vi "Basement HMI.vi"() -> ()   [LabVIEW 2018]
uses:
  <vilib>/NI/Current Value Table/Type Defs/Single Tag.ctl
  <vilib>/NI/Current Value Table/Type Defs/Data Types.ctl
  <vilib>/Utility/sysdir.llb/System Directory Type.ctl
  <vilib>/NI/Current Value Table/DataTypes/Boolean_Write.vi
  <vilib>/NI/STM/TCP/Read Meta Data (TCP Ref).vi
  <vilib>/NI/STM/TCP/Get Connection Reference (TCP).vi
  <vilib>/NI/Current Value Table/Type to Enum.vi
  <vilib>/NI/Current Value Table/DataTypes/Boolean_Type To Enum.vi
  <vilib>/NI/AMC/Read Termination Message.vi
  <vilib>/NI/AMC/Create Single Message.vi
  <vilib>/NI/AMC/Update Message Routing Info.vi
  <vilib>/NI/STM/TCP/Read Meta Data (TCP Clst).vi
  <vilib>/NI/Current Value Table/FGVs/CVT Globals.vi
  <vilib>/NI/Current Value Table/FGVs/Tag Memory.vi
  <vilib>/NI/Current Value Table/Memory Block.vi
  <vilib>/NI/Current Value Table/DataTypes/Boolean_Memory Block.vi
  <vilib>/NI/AMC/Globals.vi
  <vilib>/NI/STM/TCP/Write Message (TCP).vi
  <vilib>/NI/AMC/Send Message.vi
  <vilib>/NI/AMC/AMC.lvlib
  <vilib>/NI/STM/NI STM.lvlib
  <vilib>/NI/Current Value Table/Current Value Table.lvlib
panel:
  out "status":string
  in  "Tab Control":T1(tab)
  in  "Reset Alarms":bool
  in  "Run":bool
  in  "exit":bool
  in  "Alarms":i32(listbox)=-1
  out "PLC Model":string
  out "PLC Firmware":string
  out "PLC Sweep Time":dbl format="%#.4f"
  out "Circulator 3":bool caption="Circulator P3"
  out "Chilled Water In":dbl(knob) scale=0.0..25.0
  out "Chilled Water Out":dbl(knob) scale=0.0..25.0
  out "Chilled Water Valve":dbl(slide) scale=0.0..100.0
  out "Tempered Water In":dbl(knob) scale=15.0..35.0
  out "Tempered Water Out":dbl(knob) scale=15.0..35.0
  out "Tempered Water Valve":dbl(slide) scale=0.0..100.0
  out "Circulator 1":bool caption="Circulator P1"
  out "Circulator 2":bool caption="Circulator P2"
  out "Boiler Water In":dbl(knob) scale=10.0..100.0
  out "Boiler Water Out":dbl(knob) scale=10.0..100.0
  out "Boiler Water Valve":dbl(slide) scale=0.0..100.0
  out "Oxide Left To Dose":dbl format="%#.1f"
  out "OxideDose Indicate 1":bool caption="Oxide Dosing"
  in  "Oxide grams to Add 1":dbl=2.0 caption="Oxide grams to Add" min=-1000.0 max=1000.0 step=0.1
  in  "Dose Extra Oxide 1":bool caption="Dose Extra Oxide"
  out "FlowToOxSys 1":dbl(slide) caption="Flow To Oxide Sys" scale=0.0..12.0 scale format="%.1f"
  out "Chilled Water Injection 1":u8(slide) caption="Chilled Water Injection" scale=0.0..100.0
  out "Tempered Water Injection 1":u8(slide) caption="Tempered Water Injection" scale=0.0..100.0
  in  "T Setpoint 1":dbl=15.0 caption="T Setpoint" min=15.0 max=28.0 step=0.5
  in  "Flow to Oxide 1":dbl=2.0 caption="Flow to Oxide" min=2.0 max=12.0 step=0.1
  in  "Enable Oxide System 1":bool caption="Enable Oxide System"
  in  "Enable T Control 1":bool caption="Enable T Control"
  out "T °C 1":dbl(slide) caption="T °C" scale=0.0..30.0
  out "Proc4MainPumpInd 2":bool
  out "DI Flow Rate 1":u8(slide) caption="DI Flow Rate" scale=0.0..75.0
  out "Liters DI Added 1":dbl caption="Liters DI Added" format="%.1f"
  in  "DI Add Volume 1":dbl caption="DI Add Volume" min=0.0 max=500.0 step=0.25
  in  "Add DI water 1":bool caption="Add DI Water"
  in  "Drain System to Tree 1":bool caption="Drain System to Tree"
  out "Plating Tanks In Use South PE":bool
  in  "Enable Main Pump":bool
  out "Tank 1":dbl(slide) caption="Tank" scale=0.0..1000.0
  out "Oxide Pump":bool
  out "Oxide Pump 2":bool
  out "FlowToOxSys 2":dbl(slide) caption="Flow To Oxide Sys" scale=0.0..12.0 scale format="%.1f"
  in  "DI Add Volume 2":dbl caption="DI Add Volume"
  in  "Add DI water 2":bool caption="Add DI Water"
  out "Chilled Water Injection2":u8(slide) caption="Chilled Water Injection" scale=0.0..100.0
  out "Tempered Water Injection2":u8(slide) caption="Tempered Water Injection" scale=0.0..100.0
  out "Proc2MainPumpInd":bool
  in  "T Setpoint 2":dbl caption="T Setpoint"
  out "DI Flow Rate 2":u8(slide) caption="DI Flow Rate" scale=0.0..100.0
  in  "Flow to Oxide 2":dbl caption="Flow to Oxide"
  in  "Enable Oxide System 2":bool caption="Enable Oxide System"
  in  "Enable T Control 2":bool caption="Enable T Control"
  out "Liters DI Added 2":dbl caption="Liters DI Added" format="%.1f"
  out "T °C 2":dbl(slide) caption="T °C" scale=0.0..30.0
  out "Plating Tanks In Use S. PE":bool
  in  "Drain System to Tree 2":bool caption="Drain System to Tree"
  in  "Enable Main Pump 2":bool caption="Enable Main Pump"
  out "Tank 2":dbl(slide) scale=0.0..1000.0
  out "Oxide Pump 3":bool
  in  "Flow to Oxide 3":dbl=2.0 caption="Flow to Oxide" min=2.0 max=12.0 step=0.10000000149011612 format="%.1f"
  in  "Enable Oxide System 3":bool caption="Enable Oxide System"
  out "Proc2MainPumpInd 2":bool
  in  "DI Add Volume 3":dbl caption="DI Add Volume"
  in  "Add DI water 3":bool caption="Add DI Water"
  in  "T Setpoint 3":dbl=15.0 caption="T Setpoint" min=15.0 max=85.0 step=0.1
  in  "Enable T Control 3":bool caption="Enable T Control"
  out "Chilled Water Injection2 3":u8(slide) caption="Boiler Water Injection" scale=0.0..100.0
  out "Chilled Water Injection2 2":u8(slide) caption="Chilled Water Injection" scale=0.0..100.0
  out "Tempered Water Injection2 2":u8(slide) caption="Tempered Water Injection" scale=0.0..100.0
  out "T °C 3":dbl(slide) caption="T °C" scale=0.0..100.0
  out "Tank 3":dbl(slide) scale=0.0..1000.0
  out "DI Flow Rate 3":u8(slide) caption="DI Flow Rate" scale=0.0..100.0
  out "Liters DI Added 3":dbl caption="Liters DI Added" format="%.1f"
  in  "Drain System to Tree 3":bool caption="Drain System to Tree"
  in  "Enable Main Pump 3":bool caption="Enable Main Pump"
  out "Plating Tanks In Use S. PE 3":bool caption="Plating Tanks In Use S. PE"
  out "FlowToOxSys 3":dbl(slide) caption="Flow To Oxide Sys" scale=0.0..12.0 scale format="%.1f"
  in  "Pump Speed 4":dbl=5.0 caption="Pump Speed" min=5.0 max=100.0 step=0.5
  out "Proc4MainPumpInd":bool
  out "DI Flow Rate 4":u8(slide) caption="DI Flow Rate" scale=0.0..75.0
  out "Liters DI Added 4":dbl caption="Liters DI Added" format="%.1f"
  in  "DI Add Volume 4":dbl caption="DI Add Volume"
  in  "Add DI water 4":bool caption="Add DI Water"
  in  "Drain System to Tree 4":bool caption="Drain System to Tree"
  in  "Enable Main Pump 4":bool caption="Enable Main Pump"
  out "Tank 340":dbl(slide) scale=0.0..1500.0
  # "°C"
  # "°C"
  # "°C"
  # "°C"
  # "°C"
  # "°C"
  # "T 341"
  # "T 345"
  # "T 349"
  # "%"
  # "T 340"
  # "L"
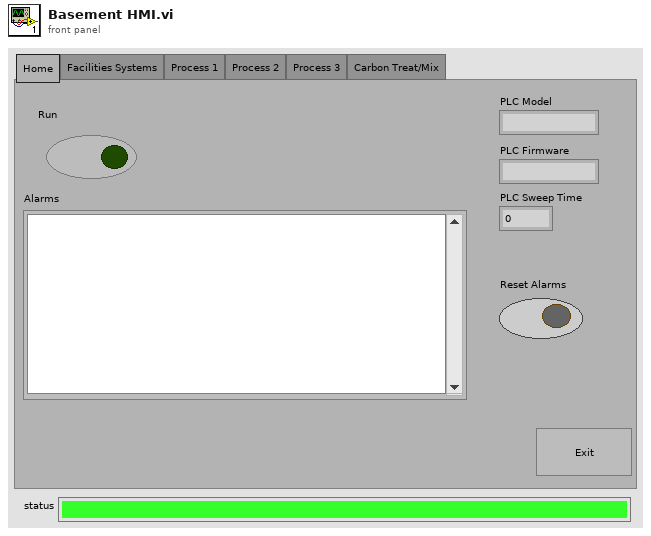
[diagram p1: front panel]
types:
  T1 = enum32{"Home", "Facilities Systems", "Process 1", "Process 2", "Process 3", "Carbon Treat/Mix"}
  T2 = typedef "System Directory Type.ctl" = i32
  T3 = typedef "Current Value Table.lvlib/Single Tag.ctl" = cluster{"Data Type":T4, "Name":string, "Value":string, "Description":string}
  T4 = typedef "Current Value Table.lvlib/Data Types.ctl" = enum16{"Double", "Single", "I64", "I32", "I16", "I8", "U64", "U32", "U16", "U8", "String", "Boolean", "Array of U8", "Array of U16", "Array of U32", "Array of U64", "Array of I64", "Array of I32", "Array of I16", "Array of I8", "Array of Double", "Array of Single", "Array of Boolean", "Array of String"}
  T5 = typedef "tae_AlarmTagConfiguration.ctl" = cluster{"Name":string, "DataType":T6, "Alarm Configuration":T7}
  T6 = typedef "cvt_Data Types.ctl" = enum16{"Bool", "U8", "I32", "Double", "String", "Enum"}
  T7 = typedef "tae_AlarmConfiguration.ctl" = cluster{"Type":T8, "High Level":dbl, "Low Level":dbl, "Hysterisis":dbl, "Deadband":dbl}
  T8 = typedef "tae_AlarmType.ctl" = enum32{"Bool True", "Bool False", "Over Limit", "Under Limit", "Out-of-Range", "Enum Equal", "Enum Not Equal"}
  T9 = typedef "Current Value Table.lvlib/File Format.ctl" = cluster{"Tags":T3[], "Group Listings":T10[]}
  T10 = typedef "Current Value Table.lvlib/Tag Grouping set.ctl" = cluster{"Group":string, "Tag Names":string[]}
  T11 = typedef "tae_AlarmCommOut.ctl" = refnum<queue>
  T12 = typedef "tae_AlarmTagList.ctl" = T5[]
  T13 = typedef "AMC.lvlib/Message Queue.ctl" = refnum<queue>
  T14 = typedef "NI STM.lvlib/TCP Connection Info.ctl" = cluster{"connection ID":refnum<k5>, "meta data":T15[]}
  T15 = typedef "NI STM.lvlib/MetaDataElement.ctl" = string
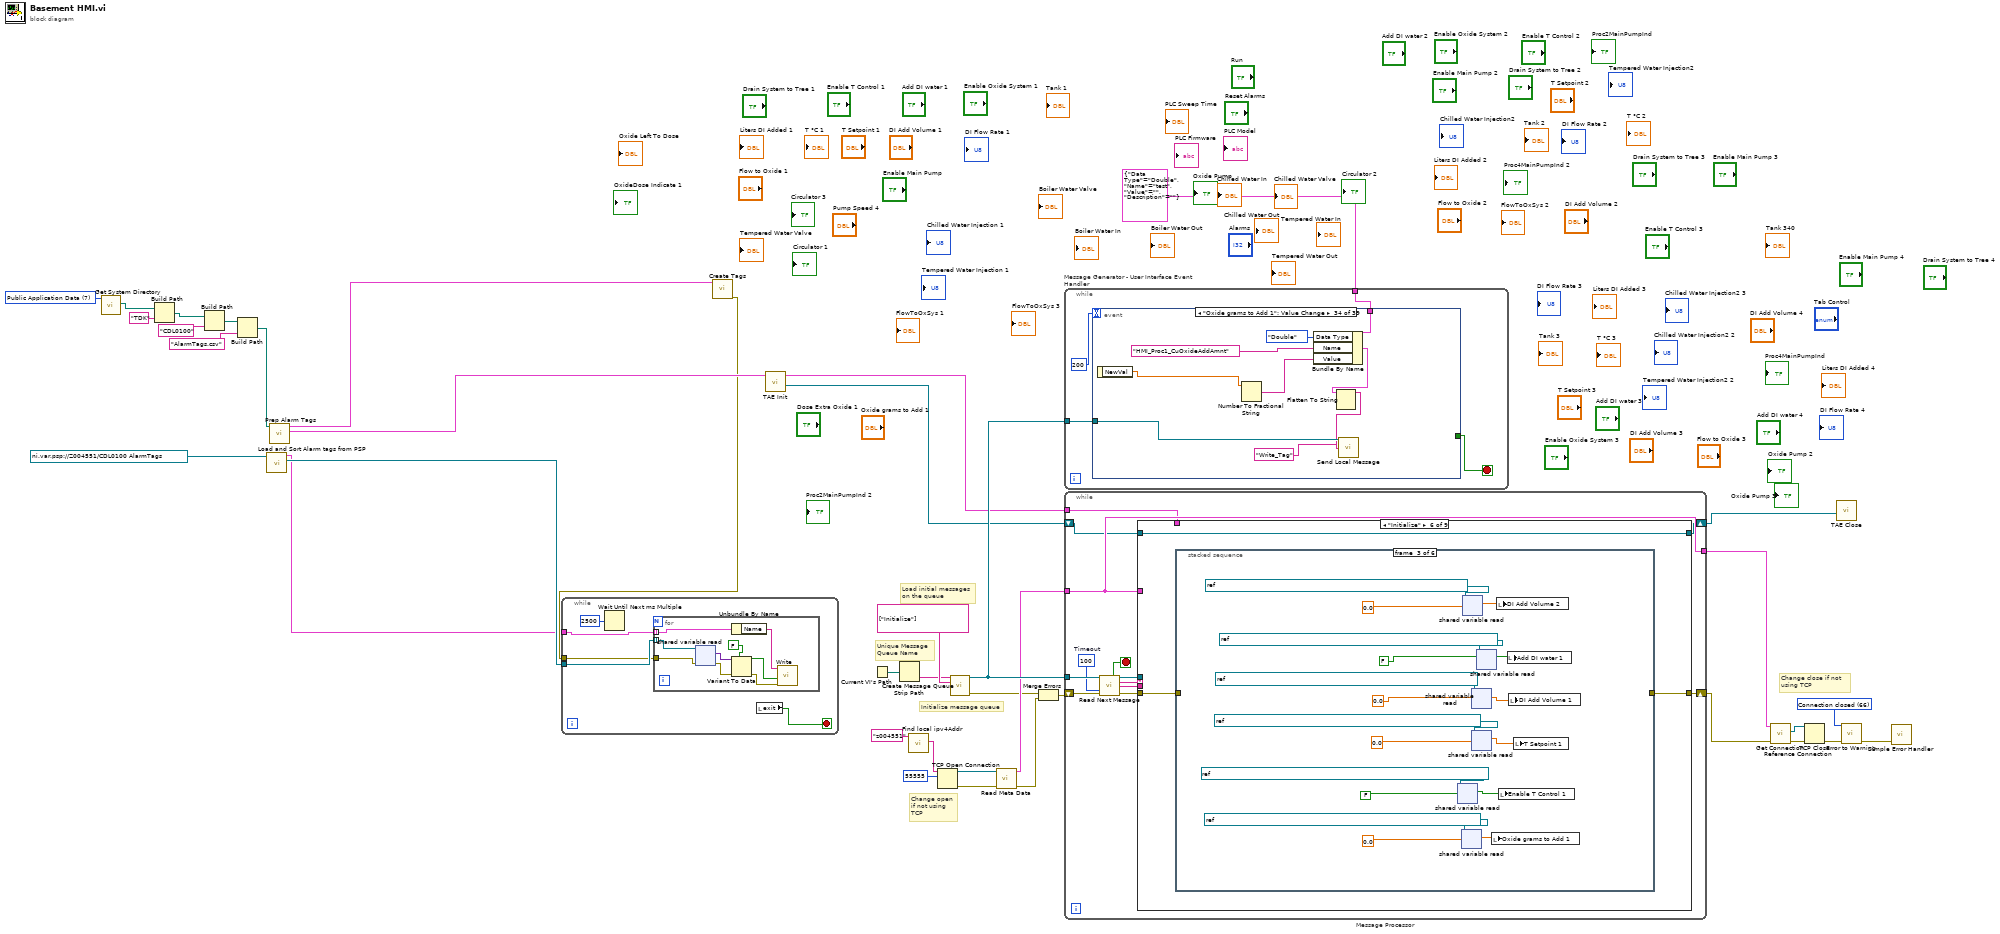
[diagram p0: block diagram]
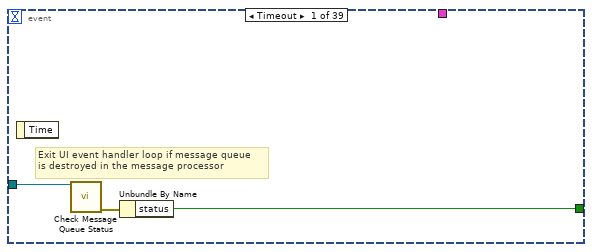
[diagram p2: hidden frame]
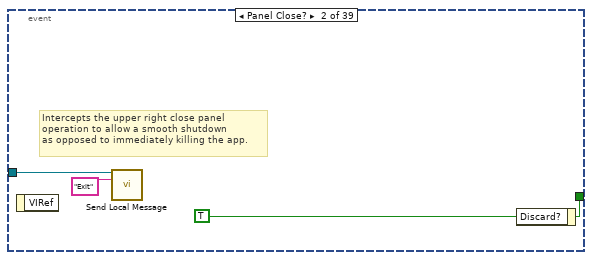
[diagram p3: hidden frame]
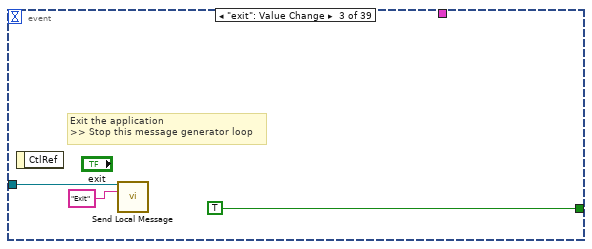
[diagram p4: hidden frame]
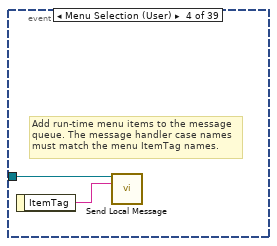
[diagram p5: hidden frame]
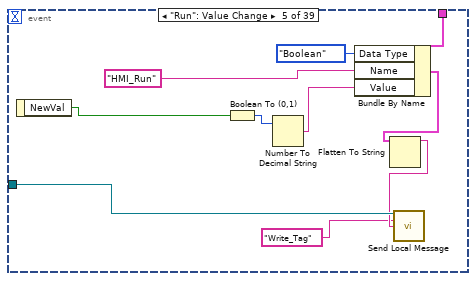
[diagram p6: hidden frame]
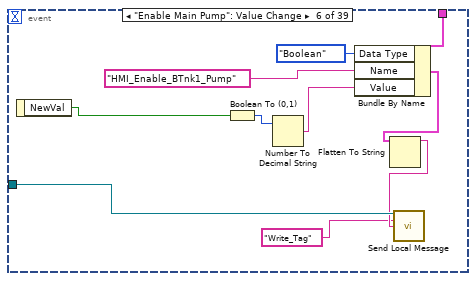
[diagram p7: hidden frame]
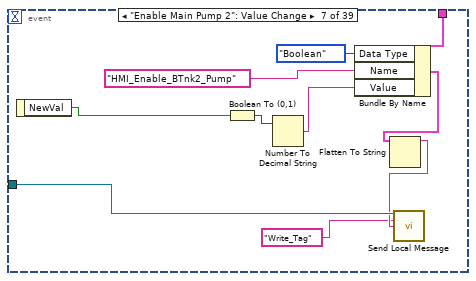
[diagram p8: hidden frame]
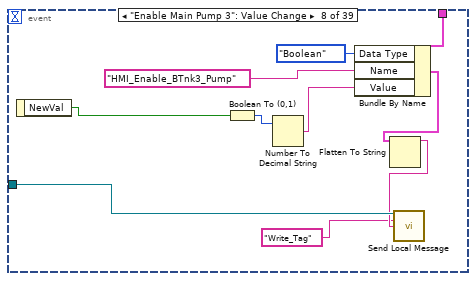
[diagram p9: hidden frame]
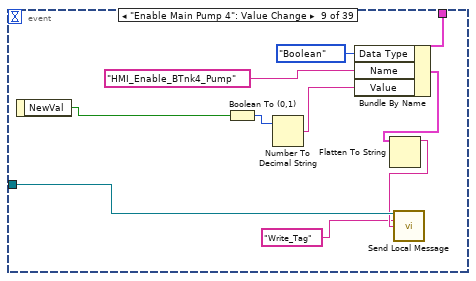
[diagram p10: hidden frame]
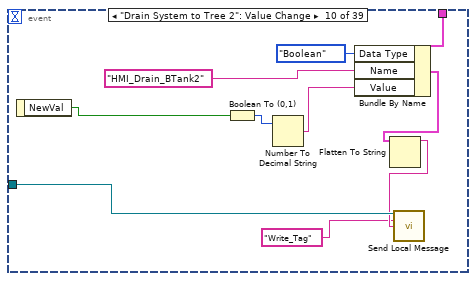
[diagram p11: hidden frame]
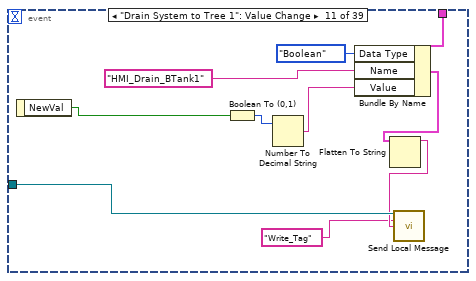
[diagram p12: hidden frame]
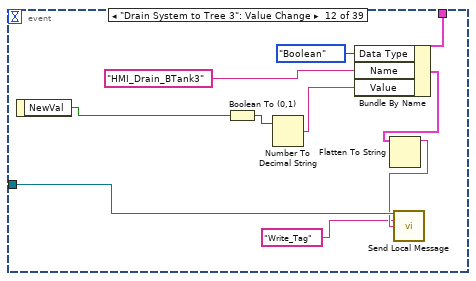
[diagram p13: hidden frame]
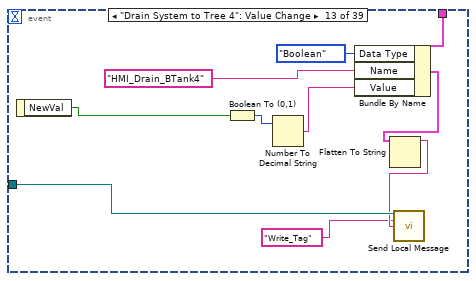
[diagram p14: hidden frame]
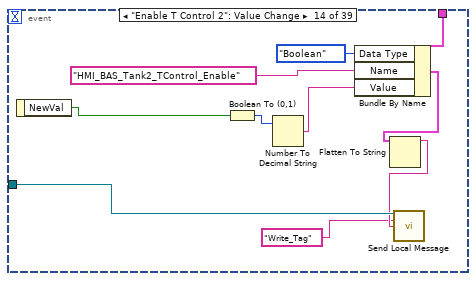
[diagram p15: hidden frame]
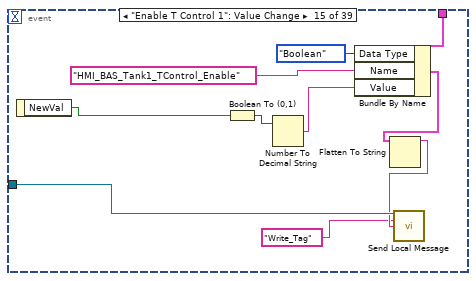
[diagram p16: hidden frame]
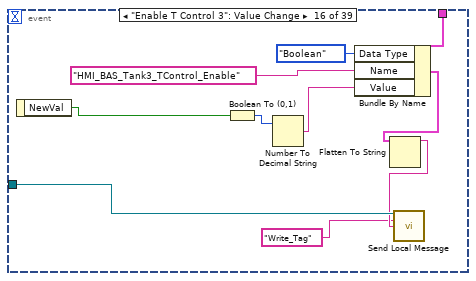
[diagram p17: hidden frame]
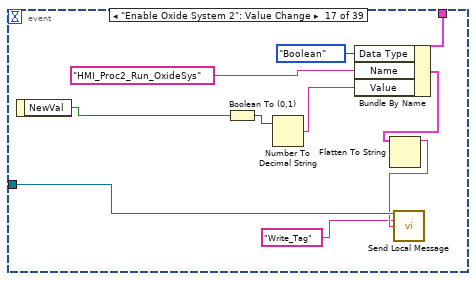
[diagram p18: hidden frame]
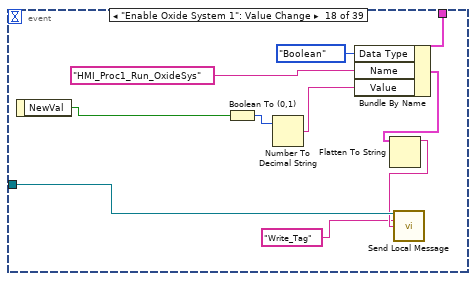
[diagram p19: hidden frame]
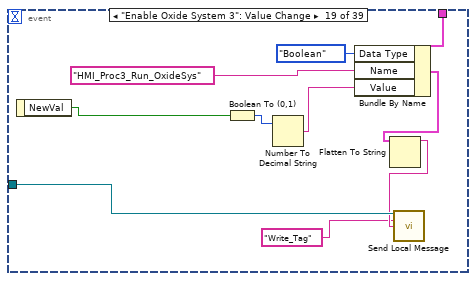
[diagram p20: hidden frame]
diagram:
  w8 = T2 7 items=["User Home"=0, "User Desktop"=1, "User Documents"=2, "User Application Data"=3, "User Preferences"=4, "User Temporary"=5, "Public Documents"=6, "Public Application Data"=7, "Public Preferences"=8, "Public Cache"=13, "System Core Libraries"=9, "System Installed Libraries"=10, "Application Files"=11, "Boot Volume Root"=12] ("system directory type")
  w28 = 66 items=["No Error", "Argument Error", "Memory Full", "Out of Zone", "End of File", "File Already Open", "Generic File IO Error", "File Not Found", "File Permission Error", "Disk Full", "Duplicate Path", "Too Many Files Open", "Not Enabled", "Resource File Not Found", "Cannot Add Resource", "Resource Not Found", "Image Not Found", "Image Memory Error", "Pen Does Not Exist", "Config Bad Type", "Config Token Not Found", "Config Parse Error", "Config Memory Error", "Bad External Code Format", "Bad External Code Offset", "External Code Not Present", "Null Window", "Destroy Window Mixup", "Null Menu", "Print Aborted", "Bad Print Record", "Print Driver Error", "Windows Error During Print", "Memory Error During Print", "Print Dialog Error", "Generic Print Error", "Invalid Device Refnum", "Device Not Found", "Device Parameter Error", "Device Unit Error", "Can't Open Device", "Device Call Aborted", "Generic Error", "Cancelled By User", "Object ID Too Low", "Object ID Too High", "Object Not In Heap", "Unknown Heap", "Bad DefProc ID", "DefProc Not In Table", "Message Out Of Range", "Null Method", "Unknown Message", "Manager Call Not Supported", "Bad address", "Connection In progress", "Connection timed out", "Connection is already in progress", "Network attribute not supported", "Network error", "Address in use", "System out of memory", "Connection aborted", "Connection refused", "Connection is not connected", "Connection is already connected", "Connection closed", "Initialize error (interapplication manager)", "Bad occurrence", "Wait on unbound occurrence handler", "Occurrence queue overflow", "Bad path", "Semaphore not signaled", "Unrecognized type (interapplication manager)"] ("1st Error to Convert")
  # "Change close if not using TCP"
  # "Change open if not using TCP"
  # "Initialize message queue"
  # "Unique Message\nQueue Name"
  # "Load initial messages\non the queue"
  n1 = call <vilib>:"Get System Directory.vi"("system directory type"=w8) -> ("system directory"=w7:path)  [unwired: 10 in]
  n2 = Build Path(base path=w7, name or relative path="TDK") -> (appended path=w5:path)
  n3 = Build Path(base path=w5, name or relative path="CDL0100") -> (appended path=w3:path)
  n4 = Build Path(base path=w3, name or relative path="AlarmTags.csv") -> (appended path=w1:path)
  n5 = call "Load and Sort Alarm tags from PSP.vi"("Refnum in"=refnum<k21> "ni.var.psp://Z004551/CDL0100 AlarmTags") -> ("Array 2"=w15:refnum<k21>[], "Array"=w9:T3[])  [unwired: 9 in]
  n6 = call "Prep Alarm Tags.vi"("Alarm Tag Description path"=w1) -> ("Alarm Array"=w16:T5[], "CVT Tags to Create"=w14:T9)  [unwired: 9 in]
  n7 = call <vilib>:"Create Tags.vi"("CVT Tags to Create"=w14) -> ("error out"=w13:errorcluster)  [unwired: 10 in]
  n8 = while {
    tunnel: w15 -> [w41]
    tunnel: w13 -> [w40]
    tunnel: w9 -> [w39]
    stop <- w43 stop-if-true
    n9 = Wait Until Next ms Multiple(millisecond multiple=u32 2500) -> ()  [unwired: 1 out]
    n10 = for {
      tunnel: w41 -> [w52] mode=indexing
      tunnel: w40 -> [w46]
      tunnel: w39 -> [w44] mode=indexing
      n11 = shared-variable-read(w52, w46) -> (w47:errorcluster, w51:variant)  [unwired: 2 out]
      n12 = Unbundle By Name(w44) -> ("Name"=w45:string)
      n13 = Variant To Data(error in=w47, type=FALSE, Variant=w51) -> (data=w49:bool, error out=w48:errorcluster)
      n14 = call-poly <vilib>:"Write.vi"("error in (no error)"=w48, "Value"=w49, "Tag Name"=w45) -> ()  [unwired: 8 in, 1 out]
    }
    n15 = local read "exit"() -> (w43:bool)
  }
  n16 = call <userlib>:"TAE Init.vi"("Alarm List"=w16) -> ("queue out"=w11:T11, "Alarm List"=w10:T12)  [unwired: 8 in, 1 out]
  n17 = Current VI's Path() -> (path=w35:path)
  n18 = Strip Path(path=w35) -> (name=w37:string)  [unwired: 1 out]
  n19 = call "Find local ipv4Addr.vi"("MachineToFind"="z004551") -> ("name"=w31:string)  [unwired: 9 in, 1 out]
  n20 = TCP Open Connection(address=w31, remote port or service name=u16 55555 ("remote port")) -> (connection ID=w33:refnum<k5>, error out=w32:errorcluster)  [unwired: 1 in, 2 out]
  n21 = call <vilib>:"Create Message Queue.vi"("message queue name"=w37, "initial message names"=string[] ["Initialize"]) -> ("message queue out"=w36:T13, "error out"=w19:errorcluster)  [unwired: 12 in]
  n22 = call-poly <vilib>:"Read Meta Data.vi"("error in"=w32, "connection ID"=w33) -> ("error out"=w18:errorcluster, "connection info out"=w23:T14)  [unwired: 7 in, 1 out]
  n23 = Merge Errors(w19, w18) -> (w20:errorcluster)
  n24 = while "Message Generator - User Interface Event Handler" {
    tunnel: w36 -> [w54]
    tunnel: T3 {"Data Type"=enum."Double", "Name"="test", "Value"="", "Description"=""} ("Tag") -> [w53]
    stop <- w55 stop-if-true
    n25 = event shown="[33] \"Oxide grams to Add 1\": Value Change" {
      selector: _ -> [_ _ _ _ _ _ _ _ _ _ _ _ _ _ _ _ _ _ _ _ _ _ _ _ _ _ _ _ _ _ _ _ _ _ _ _ _ _ _]
      dyn-events: _ -> [_ _ _ _ _ _ _ _ _ _ _ _ _ _ _ _ _ _ _ _ _ _ _ _ _ _ _ _ _ _ _ _ _ _ _ _ _ _ _]
      timeout: 200 ("Event Structure Timeout (ms)") -> [_ _ _ _ _ _ _ _ _ _ _ _ _ _ _ _ _ _ _ _ _ _ _ _ _ _ _ _ _ _ _ _ _ _ _ _ _ _ _]
      tunnel: [w57 w62 TRUE ("Discard?") _ _ _ _ _ _ _ _ _ _ _ _ _ _ _ _ _ _ _ _ _ _ _ _ _ _ _ _ _ _ _ _ _ _ _ _] -> w55
      tunnel: w54 -> [w58 w60 w63 w66 w77 w87 w97 w107 w117 w127 w137 w147 w157 w167 w177 w187 w197 w207 w217 w227 w237 w247 w257 w267 w276 w285 w294 w303 w312 w321 w330 w339 w348 w357 w366 w369 _ _ w403]
      tunnel: w53 -> [_ _ _ _ w71 w81 w91 w101 w111 w121 w131 w141 w151 w161 w171 w181 w191 w201 w211 w221 w231 w241 w251 w261 w273 w282 w291 w300 w309 w318 w327 w336 w345 w354 w363 w368 _ _ _]
      event Timeout {
        # "Exit UI event handler loop if message queue\nis destroyed in the message processor"
        n26 = event-data() -> ()  [unwired: 2 out]
        n27 = call <vilib>:"Check Message Queue Status.vi"("message queue in"=w58) -> ("error out"=w59:errorcluster)  [unwired: 10 in, 4 out]
        n28 = Unbundle By Name(w59) -> ("status"=w57:bool)
      }
      event Panel Close? {
        w62 = TRUE ("Discard?")
        # "Intercepts the upper right close panel\noperation to allow a smooth shutdown\nas opposed to immediately killing the app."
        n29 = event-data() -> ()  [unwired: 2 out]
        n30 = call <vilib>:"Send Local Message.vi"("message queue in"=w60, "message name"="Exit") -> ()  [unwired: 11 in, 3 out]
        n31 = event-data("Discard?"=w62) -> ()  [unwired: 1 in, 1 out]
      }
      event "exit": Value Change {
        # "Exit the application\n>> Stop this message generator loop"
        n32 = event-data() -> ()  [unwired: 2 out]
        n33 = call <vilib>:"Send Local Message.vi"("message queue in"=w63, "message name"="Exit") -> ()  [unwired: 11 in, 3 out]
      }
      event Menu Selection (User) {
        # "Add run-time menu items to the message\nqueue. The message handler case names must match the menu ItemTag names."
        n34 = event-data() -> ("ItemTag"=w67:string)  [unwired: 1 out]
        n35 = call <vilib>:"Send Local Message.vi"("message queue in"=w66, "message name"=w67) -> ()  [unwired: 11 in, 3 out]
      }
      event "Run": Value Change {
        n36 = event-data() -> ("NewVal"=w72:bool)  [unwired: 1 out]
        n37 = Boolean To (0,1)(Boolean=w72) -> (0, 1=w76:i16)
        n38 = Number To Decimal String(number=w76) -> (decimal integer string=w75:string)  [unwired: 1 in]
        n39 = Bundle By Name(cluster=w71, "Data Type"=Data_Types."Boolean", "Name"="HMI_Run", "Value"=w75) -> (w70:T3)
        n40 = Flatten To String(anything=w70) -> (data string=w69:string)  [unwired: 3 in, 2 out]
        n41 = call <vilib>:"Send Local Message.vi"("message queue in"=w77, "message name"="Write_Tag", "message value"=w69) -> ()  [unwired: 10 in, 3 out]
      }
      event "Enable Main Pump": Value Change {
        n42 = event-data() -> ("NewVal"=w82:bool)  [unwired: 1 out]
        n43 = Boolean To (0,1)(Boolean=w82) -> (0, 1=w86:i16)
        n44 = Number To Decimal String(number=w86) -> (decimal integer string=w85:string)  [unwired: 1 in]
        n45 = Bundle By Name(cluster=w81, "Data Type"=Data_Types."Boolean", "Name"="HMI_Enable_BTnk1_Pump", "Value"=w85) -> (w80:T3)
        n46 = Flatten To String(anything=w80) -> (data string=w79:string)  [unwired: 3 in, 2 out]
        n47 = call <vilib>:"Send Local Message.vi"("message queue in"=w87, "message name"="Write_Tag", "message value"=w79) -> ()  [unwired: 10 in, 3 out]
      }
      event "Enable Main Pump 2": Value Change {
        n48 = event-data() -> ("NewVal"=w92:bool)  [unwired: 1 out]
        n49 = Boolean To (0,1)(Boolean=w92) -> (0, 1=w96:i16)
        n50 = Number To Decimal String(number=w96) -> (decimal integer string=w95:string)  [unwired: 1 in]
        n51 = Bundle By Name(cluster=w91, "Data Type"=Data_Types."Boolean", "Name"="HMI_Enable_BTnk2_Pump", "Value"=w95) -> (w90:T3)
        n52 = Flatten To String(anything=w90) -> (data string=w89:string)  [unwired: 3 in, 2 out]
        n53 = call <vilib>:"Send Local Message.vi"("message queue in"=w97, "message name"="Write_Tag", "message value"=w89) -> ()  [unwired: 10 in, 3 out]
      }
      event "Enable Main Pump 3": Value Change {
        n54 = event-data() -> ("NewVal"=w102:bool)  [unwired: 1 out]
        n55 = Boolean To (0,1)(Boolean=w102) -> (0, 1=w106:i16)
        n56 = Number To Decimal String(number=w106) -> (decimal integer string=w105:string)  [unwired: 1 in]
        n57 = Bundle By Name(cluster=w101, "Data Type"=Data_Types."Boolean", "Name"="HMI_Enable_BTnk3_Pump", "Value"=w105) -> (w100:T3)
        n58 = Flatten To String(anything=w100) -> (data string=w99:string)  [unwired: 3 in, 2 out]
        n59 = call <vilib>:"Send Local Message.vi"("message queue in"=w107, "message name"="Write_Tag", "message value"=w99) -> ()  [unwired: 10 in, 3 out]
      }
      event "Enable Main Pump 4": Value Change {
        n60 = event-data() -> ("NewVal"=w112:bool)  [unwired: 1 out]
        n61 = Boolean To (0,1)(Boolean=w112) -> (0, 1=w116:i16)
        n62 = Number To Decimal String(number=w116) -> (decimal integer string=w115:string)  [unwired: 1 in]
        n63 = Bundle By Name(cluster=w111, "Data Type"=Data_Types."Boolean", "Name"="HMI_Enable_BTnk4_Pump", "Value"=w115) -> (w110:T3)
        n64 = Flatten To String(anything=w110) -> (data string=w109:string)  [unwired: 3 in, 2 out]
        n65 = call <vilib>:"Send Local Message.vi"("message queue in"=w117, "message name"="Write_Tag", "message value"=w109) -> ()  [unwired: 10 in, 3 out]
      }
      event "Drain System to Tree 2": Value Change {
        n66 = event-data() -> ("NewVal"=w122:bool)  [unwired: 1 out]
        n67 = Boolean To (0,1)(Boolean=w122) -> (0, 1=w126:i16)
        n68 = Number To Decimal String(number=w126) -> (decimal integer string=w125:string)  [unwired: 1 in]
        n69 = Bundle By Name(cluster=w121, "Data Type"=Data_Types."Boolean", "Name"="HMI_Drain_BTank2", "Value"=w125) -> (w120:T3)
        n70 = Flatten To String(anything=w120) -> (data string=w119:string)  [unwired: 3 in, 2 out]
        n71 = call <vilib>:"Send Local Message.vi"("message queue in"=w127, "message name"="Write_Tag", "message value"=w119) -> ()  [unwired: 10 in, 3 out]
      }
      event "Drain System to Tree 1": Value Change {
        n72 = event-data() -> ("NewVal"=w132:bool)  [unwired: 1 out]
        n73 = Boolean To (0,1)(Boolean=w132) -> (0, 1=w136:i16)
        n74 = Number To Decimal String(number=w136) -> (decimal integer string=w135:string)  [unwired: 1 in]
        n75 = Bundle By Name(cluster=w131, "Data Type"=Data_Types."Boolean", "Name"="HMI_Drain_BTank1", "Value"=w135) -> (w130:T3)
        n76 = Flatten To String(anything=w130) -> (data string=w129:string)  [unwired: 3 in, 2 out]
        n77 = call <vilib>:"Send Local Message.vi"("message queue in"=w137, "message name"="Write_Tag", "message value"=w129) -> ()  [unwired: 10 in, 3 out]
      }
      event "Drain System to Tree 3": Value Change {
        n78 = event-data() -> ("NewVal"=w142:bool)  [unwired: 1 out]
        n79 = Boolean To (0,1)(Boolean=w142) -> (0, 1=w146:i16)
        n80 = Number To Decimal String(number=w146) -> (decimal integer string=w145:string)  [unwired: 1 in]
        n81 = Bundle By Name(cluster=w141, "Data Type"=Data_Types."Boolean", "Name"="HMI_Drain_BTank3", "Value"=w145) -> (w140:T3)
        n82 = Flatten To String(anything=w140) -> (data string=w139:string)  [unwired: 3 in, 2 out]
        n83 = call <vilib>:"Send Local Message.vi"("message queue in"=w147, "message name"="Write_Tag", "message value"=w139) -> ()  [unwired: 10 in, 3 out]
      }
      event "Drain System to Tree 4": Value Change {
        n84 = event-data() -> ("NewVal"=w152:bool)  [unwired: 1 out]
        n85 = Boolean To (0,1)(Boolean=w152) -> (0, 1=w156:i16)
        n86 = Number To Decimal String(number=w156) -> (decimal integer string=w155:string)  [unwired: 1 in]
        n87 = Bundle By Name(cluster=w151, "Data Type"=Data_Types."Boolean", "Name"="HMI_Drain_BTank4", "Value"=w155) -> (w150:T3)
        n88 = Flatten To String(anything=w150) -> (data string=w149:string)  [unwired: 3 in, 2 out]
        n89 = call <vilib>:"Send Local Message.vi"("message queue in"=w157, "message name"="Write_Tag", "message value"=w149) -> ()  [unwired: 10 in, 3 out]
      }
      event "Enable T Control 2": Value Change {
        n90 = event-data() -> ("NewVal"=w162:bool)  [unwired: 1 out]
        n91 = Boolean To (0,1)(Boolean=w162) -> (0, 1=w166:i16)
        n92 = Number To Decimal String(number=w166) -> (decimal integer string=w165:string)  [unwired: 1 in]
        n93 = Bundle By Name(cluster=w161, "Data Type"=Data_Types."Boolean", "Name"="HMI_BAS_Tank2_TControl_Enable", "Value"=w165) -> (w160:T3)
        n94 = Flatten To String(anything=w160) -> (data string=w159:string)  [unwired: 3 in, 2 out]
        n95 = call <vilib>:"Send Local Message.vi"("message queue in"=w167, "message name"="Write_Tag", "message value"=w159) -> ()  [unwired: 10 in, 3 out]
      }
      event "Enable T Control 1": Value Change {
        n96 = event-data() -> ("NewVal"=w172:bool)  [unwired: 1 out]
        n97 = Boolean To (0,1)(Boolean=w172) -> (0, 1=w176:i16)
        n98 = Number To Decimal String(number=w176) -> (decimal integer string=w175:string)  [unwired: 1 in]
        n99 = Bundle By Name(cluster=w171, "Data Type"=Data_Types."Boolean", "Name"="HMI_BAS_Tank1_TControl_Enable", "Value"=w175) -> (w170:T3)
        n100 = Flatten To String(anything=w170) -> (data string=w169:string)  [unwired: 3 in, 2 out]
        n101 = call <vilib>:"Send Local Message.vi"("message queue in"=w177, "message name"="Write_Tag", "message value"=w169) -> ()  [unwired: 10 in, 3 out]
      }
      event "Enable T Control 3": Value Change {
        n102 = event-data() -> ("NewVal"=w182:bool)  [unwired: 1 out]
        n103 = Boolean To (0,1)(Boolean=w182) -> (0, 1=w186:i16)
        n104 = Number To Decimal String(number=w186) -> (decimal integer string=w185:string)  [unwired: 1 in]
        n105 = Bundle By Name(cluster=w181, "Data Type"=Data_Types."Boolean", "Name"="HMI_BAS_Tank3_TControl_Enable", "Value"=w185) -> (w180:T3)
        n106 = Flatten To String(anything=w180) -> (data string=w179:string)  [unwired: 3 in, 2 out]
        n107 = call <vilib>:"Send Local Message.vi"("message queue in"=w187, "message name"="Write_Tag", "message value"=w179) -> ()  [unwired: 10 in, 3 out]
      }
      event "Enable Oxide System 2": Value Change {
        n108 = event-data() -> ("NewVal"=w192:bool)  [unwired: 1 out]
        n109 = Boolean To (0,1)(Boolean=w192) -> (0, 1=w196:i16)
        n110 = Number To Decimal String(number=w196) -> (decimal integer string=w195:string)  [unwired: 1 in]
        n111 = Bundle By Name(cluster=w191, "Data Type"=Data_Types."Boolean", "Name"="HMI_Proc2_Run_OxideSys", "Value"=w195) -> (w190:T3)
        n112 = Flatten To String(anything=w190) -> (data string=w189:string)  [unwired: 3 in, 2 out]
        n113 = call <vilib>:"Send Local Message.vi"("message queue in"=w197, "message name"="Write_Tag", "message value"=w189) -> ()  [unwired: 10 in, 3 out]
      }
      event "Enable Oxide System 1": Value Change {
        n114 = event-data() -> ("NewVal"=w202:bool)  [unwired: 1 out]
        n115 = Boolean To (0,1)(Boolean=w202) -> (0, 1=w206:i16)
        n116 = Number To Decimal String(number=w206) -> (decimal integer string=w205:string)  [unwired: 1 in]
        n117 = Bundle By Name(cluster=w201, "Data Type"=Data_Types."Boolean", "Name"="HMI_Proc1_Run_OxideSys", "Value"=w205) -> (w200:T3)
        n118 = Flatten To String(anything=w200) -> (data string=w199:string)  [unwired: 3 in, 2 out]
        n119 = call <vilib>:"Send Local Message.vi"("message queue in"=w207, "message name"="Write_Tag", "message value"=w199) -> ()  [unwired: 10 in, 3 out]
      }
      event "Enable Oxide System 3": Value Change {
        n120 = event-data() -> ("NewVal"=w212:bool)  [unwired: 1 out]
        n121 = Boolean To (0,1)(Boolean=w212) -> (0, 1=w216:i16)
        n122 = Number To Decimal String(number=w216) -> (decimal integer string=w215:string)  [unwired: 1 in]
        n123 = Bundle By Name(cluster=w211, "Data Type"=Data_Types."Boolean", "Name"="HMI_Proc3_Run_OxideSys", "Value"=w215) -> (w210:T3)
        n124 = Flatten To String(anything=w210) -> (data string=w209:string)  [unwired: 3 in, 2 out]
        n125 = call <vilib>:"Send Local Message.vi"("message queue in"=w217, "message name"="Write_Tag", "message value"=w209) -> ()  [unwired: 10 in, 3 out]
      }
      event "Add DI water 2": Value Change {
        n126 = event-data() -> ("NewVal"=w222:bool)  [unwired: 1 out]
        n127 = Boolean To (0,1)(Boolean=w222) -> (0, 1=w226:i16)
        n128 = Number To Decimal String(number=w226) -> (decimal integer string=w225:string)  [unwired: 1 in]
        n129 = Bundle By Name(cluster=w221, "Data Type"=Data_Types."Boolean", "Name"="HMI_BAS_Proc2_AddDIVolume", "Value"=w225) -> (w220:T3)
        n130 = Flatten To String(anything=w220) -> (data string=w219:string)  [unwired: 3 in, 2 out]
        n131 = call <vilib>:"Send Local Message.vi"("message queue in"=w227, "message name"="Write_Tag", "message value"=w219) -> ()  [unwired: 10 in, 3 out]
      }
      event "Add DI water 1": Value Change {
        n132 = event-data() -> ("NewVal"=w232:bool)  [unwired: 1 out]
        n133 = Boolean To (0,1)(Boolean=w232) -> (0, 1=w236:i16)
        n134 = Number To Decimal String(number=w236) -> (decimal integer string=w235:string)  [unwired: 1 in]
        n135 = Bundle By Name(cluster=w231, "Data Type"=Data_Types."Boolean", "Name"="HMI_BAS_Proc1_AddDIVolume", "Value"=w235) -> (w230:T3)
        n136 = Flatten To String(anything=w230) -> (data string=w229:string)  [unwired: 3 in, 2 out]
        n137 = call <vilib>:"Send Local Message.vi"("message queue in"=w237, "message name"="Write_Tag", "message value"=w229) -> ()  [unwired: 10 in, 3 out]
      }
      event "Add DI water 3": Value Change {
        n138 = event-data() -> ("NewVal"=w242:bool)  [unwired: 1 out]
        n139 = Boolean To (0,1)(Boolean=w242) -> (0, 1=w246:i16)
        n140 = Number To Decimal String(number=w246) -> (decimal integer string=w245:string)  [unwired: 1 in]
        n141 = Bundle By Name(cluster=w241, "Data Type"=Data_Types."Boolean", "Name"="HMI_BAS_Proc3_AddDIVolume", "Value"=w245) -> (w240:T3)
        n142 = Flatten To String(anything=w240) -> (data string=w239:string)  [unwired: 3 in, 2 out]
        n143 = call <vilib>:"Send Local Message.vi"("message queue in"=w247, "message name"="Write_Tag", "message value"=w239) -> ()  [unwired: 10 in, 3 out]
      }
      event "Add DI water 4": Value Change {
        n144 = event-data() -> ("NewVal"=w252:bool)  [unwired: 1 out]
        n145 = Boolean To (0,1)(Boolean=w252) -> (0, 1=w256:i16)
        n146 = Number To Decimal String(number=w256) -> (decimal integer string=w255:string)  [unwired: 1 in]
        n147 = Bundle By Name(cluster=w251, "Data Type"=Data_Types."Boolean", "Name"="HMI_BAS_Proc4_AddDIVolume", "Value"=w255) -> (w250:T3)
        n148 = Flatten To String(anything=w250) -> (data string=w249:string)  [unwired: 3 in, 2 out]
        n149 = call <vilib>:"Send Local Message.vi"("message queue in"=w257, "message name"="Write_Tag", "message value"=w249) -> ()  [unwired: 10 in, 3 out]
      }
      event "Dose Extra Oxide 1": Value Change {
        n150 = event-data() -> ("NewVal"=w262:bool)  [unwired: 1 out]
        n151 = Boolean To (0,1)(Boolean=w262) -> (0, 1=w266:i16)
        n152 = Number To Decimal String(number=w266) -> (decimal integer string=w265:string)  [unwired: 1 in]
        n153 = Bundle By Name(cluster=w261, "Data Type"=Data_Types."Boolean", "Name"="HMI_Proc1_Add_CuOxide", "Value"=w265) -> (w260:T3)
        n154 = Flatten To String(anything=w260) -> (data string=w259:string)  [unwired: 3 in, 2 out]
        n155 = call <vilib>:"Send Local Message.vi"("message queue in"=w267, "message name"="Write_Tag", "message value"=w259) -> ()  [unwired: 10 in, 3 out]
      }
      event "Flow to Oxide 2": Value Change {
        n156 = event-data() -> ("NewVal"=w269:dbl)  [unwired: 1 out]
        n157 = Number To Fractional String(number=w269) -> (F-format string=w268:string)  [unwired: 3 in]
        n158 = Bundle By Name(cluster=w273, "Data Type"=Data_Types."Double", "Name"="HMI_Proc2_OxFlow_SetPnt", "Value"=w268) -> (w272:T3)
        n159 = Flatten To String(anything=w272) -> (data string=w271:string)  [unwired: 3 in, 2 out]
        n160 = call <vilib>:"Send Local Message.vi"("message queue in"=w276, "message name"="Write_Tag", "message value"=w271) -> ()  [unwired: 10 in, 3 out]
      }
      event "Flow to Oxide 1": Value Change {
        n161 = event-data() -> ("NewVal"=w278:dbl)  [unwired: 1 out]
        n162 = Number To Fractional String(number=w278) -> (F-format string=w277:string)  [unwired: 3 in]
        n163 = Bundle By Name(cluster=w282, "Data Type"=Data_Types."Double", "Name"="HMI_Proc1_OxFlow_SetPnt", "Value"=w277) -> (w281:T3)
        n164 = Flatten To String(anything=w281) -> (data string=w280:string)  [unwired: 3 in, 2 out]
        n165 = call <vilib>:"Send Local Message.vi"("message queue in"=w285, "message name"="Write_Tag", "message value"=w280) -> ()  [unwired: 10 in, 3 out]
      }
      event "Flow to Oxide 3": Value Change {
        n166 = event-data() -> ("NewVal"=w287:dbl)  [unwired: 1 out]
        n167 = Number To Fractional String(number=w287) -> (F-format string=w286:string)  [unwired: 3 in]
        n168 = Bundle By Name(cluster=w291, "Data Type"=Data_Types."Double", "Name"="HMI_Proc3_OxFlow_SetPnt", "Value"=w286) -> (w290:T3)
        n169 = Flatten To String(anything=w290) -> (data string=w289:string)  [unwired: 3 in, 2 out]
        n170 = call <vilib>:"Send Local Message.vi"("message queue in"=w294, "message name"="Write_Tag", "message value"=w289) -> ()  [unwired: 10 in, 3 out]
      }
      event "T Setpoint 2": Value Change {
        n171 = event-data() -> ("NewVal"=w296:dbl)  [unwired: 1 out]
        n172 = Number To Fractional String(number=w296) -> (F-format string=w295:string)  [unwired: 3 in]
        n173 = Bundle By Name(cluster=w300, "Data Type"=Data_Types."Double", "Name"="HMI_BAS_TNK2_T_Setpoint", "Value"=w295) -> (w299:T3)
        n174 = Flatten To String(anything=w299) -> (data string=w298:string)  [unwired: 3 in, 2 out]
        n175 = call <vilib>:"Send Local Message.vi"("message queue in"=w303, "message name"="Write_Tag", "message value"=w298) -> ()  [unwired: 10 in, 3 out]
      }
      event "T Setpoint 3": Value Change {
        n176 = event-data() -> ("NewVal"=w305:dbl)  [unwired: 1 out]
        n177 = Number To Fractional String(number=w305) -> (F-format string=w304:string)  [unwired: 3 in]
        n178 = Bundle By Name(cluster=w309, "Data Type"=Data_Types."Double", "Name"="HMI_BAS_TNK3_T_Setpoint", "Value"=w304) -> (w308:T3)
        n179 = Flatten To String(anything=w308) -> (data string=w307:string)  [unwired: 3 in, 2 out]
        n180 = call <vilib>:"Send Local Message.vi"("message queue in"=w312, "message name"="Write_Tag", "message value"=w307) -> ()  [unwired: 10 in, 3 out]
      }
      event "DI Add Volume 2": Value Change {
        n181 = event-data() -> ("NewVal"=w314:dbl)  [unwired: 1 out]
        n182 = Number To Fractional String(number=w314) -> (F-format string=w313:string)  [unwired: 3 in]
        n183 = Bundle By Name(cluster=w318, "Data Type"=Data_Types."Double", "Name"="HMI_BAS_Proc2_DI_Setpnt", "Value"=w313) -> (w317:T3)
        n184 = Flatten To String(anything=w317) -> (data string=w316:string)  [unwired: 3 in, 2 out]
        n185 = call <vilib>:"Send Local Message.vi"("message queue in"=w321, "message name"="Write_Tag", "message value"=w316) -> ()  [unwired: 10 in, 3 out]
      }
      event "DI Add Volume 1": Value Change {
        n186 = event-data() -> ("NewVal"=w323:dbl)  [unwired: 1 out]
        n187 = Number To Fractional String(number=w323) -> (F-format string=w322:string)  [unwired: 3 in]
        n188 = Bundle By Name(cluster=w327, "Data Type"=Data_Types."Double", "Name"="HMI_BAS_Proc1_DI_Setpnt", "Value"=w322) -> (w326:T3)
        n189 = Flatten To String(anything=w326) -> (data string=w325:string)  [unwired: 3 in, 2 out]
        n190 = call <vilib>:"Send Local Message.vi"("message queue in"=w330, "message name"="Write_Tag", "message value"=w325) -> ()  [unwired: 10 in, 3 out]
      }
      event "DI Add Volume 3": Value Change {
        n191 = event-data() -> ("NewVal"=w332:dbl)  [unwired: 1 out]
        n192 = Number To Fractional String(number=w332) -> (F-format string=w331:string)  [unwired: 3 in]
        n193 = Bundle By Name(cluster=w336, "Data Type"=Data_Types."Double", "Name"="HMI_BAS_Proc3_DI_Setpnt", "Value"=w331) -> (w335:T3)
        n194 = Flatten To String(anything=w335) -> (data string=w334:string)  [unwired: 3 in, 2 out]
        n195 = call <vilib>:"Send Local Message.vi"("message queue in"=w339, "message name"="Write_Tag", "message value"=w334) -> ()  [unwired: 10 in, 3 out]
      }
      event "DI Add Volume 4": Value Change {
        n196 = event-data() -> ("NewVal"=w341:dbl)  [unwired: 1 out]
        n197 = Number To Fractional String(number=w341) -> (F-format string=w340:string)  [unwired: 3 in]
        n198 = Bundle By Name(cluster=w345, "Data Type"=Data_Types."Double", "Name"="HMI_BAS_Proc4_DI_Setpnt", "Value"=w340) -> (w344:T3)
        n199 = Flatten To String(anything=w344) -> (data string=w343:string)  [unwired: 3 in, 2 out]
        n200 = call <vilib>:"Send Local Message.vi"("message queue in"=w348, "message name"="Write_Tag", "message value"=w343) -> ()  [unwired: 10 in, 3 out]
      }
      event "Oxide grams to Add 1": Value Change {
        n201 = event-data() -> ("NewVal"=w350:dbl)  [unwired: 1 out]
        n202 = Number To Fractional String(number=w350) -> (F-format string=w349:string)  [unwired: 3 in]
        n203 = Bundle By Name(cluster=w354, "Data Type"=Data_Types."Double", "Name"="HMI_Proc1_CuOxideAddAmnt", "Value"=w349) -> (w353:T3)
        n204 = Flatten To String(anything=w353) -> (data string=w352:string)  [unwired: 3 in, 2 out]
        n205 = call <vilib>:"Send Local Message.vi"("message queue in"=w357, "message name"="Write_Tag", "message value"=w352) -> ()  [unwired: 10 in, 3 out]
      }
      event "Pump Speed 4": Value Change {
        n206 = event-data() -> ("NewVal"=w359:dbl)  [unwired: 1 out]
        n207 = Number To Fractional String(number=w359) -> (F-format string=w358:string)  [unwired: 3 in]
        n208 = Bundle By Name(cluster=w363, "Data Type"=Data_Types."Double", "Name"="HMI_BAS_Tnk4RecircPmpPcnt", "Value"=w358) -> (w362:T3)
        n209 = Flatten To String(anything=w362) -> (data string=w361:string)  [unwired: 3 in, 2 out]
        n210 = call <vilib>:"Send Local Message.vi"("message queue in"=w366, "message name"="Write_Tag", "message value"=w361) -> ()  [unwired: 10 in, 3 out]
      }
      event "Reset Alarms": Value Change {
        n211 = event-data() -> ("NewVal"=w367:bool)  [unwired: 1 out]
        n212 = case shown="True" w367 {
          tunnel: w369 -> [_ w379]
          tunnel: w367 -> [_ w374]
          tunnel: w368 -> [_ w373]
          frame False {
          }
          frame True {
            n213 = Boolean To (0,1)(Boolean=w374) -> (0, 1=w378:i16)
            n214 = Number To Decimal String(number=w378) -> (decimal integer string=w377:string)  [unwired: 1 in]
            n215 = Bundle By Name(cluster=w373, "Data Type"=Data_Types."Boolean", "Name"="HMI_Reset_Alarms", "Value"=w377) -> (w372:T3)
            n216 = Flatten To String(anything=w372) -> (data string=w371:string)  [unwired: 3 in, 2 out]
            n217 = call <vilib>:"Send Local Message.vi"("message queue in"=w379, "message name"="Write_Tag", "message value"=w371) -> ()  [unwired: 10 in, 3 out]
          }
        }
      }
      event "Flow to Oxide 2": Mouse Up {
        n218 = event-data() -> ("CtlRef"=w387:refnum<vi>)  [unwired: 8 out]
        n219 = property class="DigNum (strict)"(reference=w387) -> (reference out=w380:refnum<vi>, "Label.Text"=w386:string, "Value"=w385:dbl)  [unwired: 1 in, 1 out]
        n220 = Number To Fractional String(number=w385, precision (6)=i16 1) -> (F-format string=w384:string)  [unwired: 2 in]
        n221 = call <userlib>:"HMI Pop Up Num KP.vi"("String In"=w384, "Message In"=w386) -> ("Canceled"=w382:bool, "String Out"=w381:string)  [unwired: 8 in]
        n222 = case shown="False" w382 {
          tunnel: w381 -> [w389 _]
          tunnel: w380 -> [w390 _]
          frame False {
            n223 = Fract/Exp String To Number(string=w389) -> (number=w388:dbl)  [unwired: 3 in, 1 out]
            n224 = property class="DigNum (strict)"(reference=w390, "Val(Sgnl)"=w388) -> ()  [unwired: 1 in, 2 out]
          }
          frame True {
          }
        }
      }
      event "T Setpoint 2", "DI Add Volume 2", "DI Add Volume 4", "DI Add Volume 1", "T Setpoint 1", "Flow to Oxide 1", "Pump Speed 4", "T Setpoint 3", "DI Add Volume 3", "Flow to Oxide 3", "Oxide grams to Add 1": Mouse Up {
        n225 = event-data() -> ("CtlRef"=w398:refnum<vi>)  [unwired: 8 out]
        n226 = property class="DigNum (strict)"(reference=w398) -> (reference out=w391:refnum<vi>, "Label.Text"=w397:string, "Value"=w396:dbl)  [unwired: 1 in, 1 out]
        n227 = Number To Fractional String(number=w396, precision (6)=i16 1) -> (F-format string=w395:string)  [unwired: 2 in]
        n228 = call <userlib>:"HMI Pop Up Num KP.vi"("String In"=w395, "Message In"=w397) -> ("Canceled"=w393:bool, "String Out"=w392:string)  [unwired: 8 in]
        n229 = case shown="False" w393 {
          tunnel: w392 -> [w400 _]
          tunnel: w391 -> [w401 _]
          frame False {
            n230 = Fract/Exp String To Number(string=w400) -> (number=w399:dbl)  [unwired: 3 in, 1 out]
            n231 = property class="DigNum (strict)"(reference=w401, "Val(Sgnl)"=w399) -> ()  [unwired: 1 in, 2 out]
          }
          frame True {
          }
        }
      }
      event "Tab Control": Value Change {
        n232 = event-data() -> ()  [unwired: 7 out]
        n233 = call <vilib>:"Send Local Message.vi"("message queue in"=w403, "message name"="Initialize") -> ()  [unwired: 11 in, 3 out]
      }
    }
  }
  n234 = while "Message Processor" {
    shift-left: w20 -> [w412]
    shift-right: [w416] -> w24
    tunnel: w36 -> [w413]
    tunnel: w23 -> [w407]
    tunnel: [w407] -> w22
    shift-right: [w405] -> w12
    shift-left: w11 -> [w406]
    tunnel: w10 -> [w404]
    stop <- w415 stop-if-true
    w408 = 100  # Timeout
    n235 = call <vilib>:"Read Next Message.vi"("message queue in"=w413, "timeout (1 ms)"=w408, "error in"=w412) -> ("exit process?"=w415:bool, "message queue out"=w414:T13, "message name"=w410:string, "message value"=w409:string, "error out"=w411:errorcluster)  [unwired: 5 in, 3 out]
    n236 = case shown="\"Initialize\"" w410 {
      selector: w410 -> [_ _ w485 _ _ _ _ _ _]
      tunnel: w414 -> [_ _ _ _ _ _ w592 _ _]
      tunnel: w411 -> [w418 w424 w486 w488 w491 w494 w593 w596 w600]
      tunnel: [w418 w424 w486 errorcluster {"status"=FALSE, "code"=0, "source"=""} ("error out") w491 w493 w591 w596 w599] -> w416
      tunnel: w409 -> [_ _ _ _ _ _ _ _ w598]
      tunnel: w407 -> [_ _ _ _ _ _ _ _ w601]
      tunnel: w406 -> [w417 w423 w482 w487 w490 w492 w590 w595 w597]
      tunnel: [w417 w421 w482 w487 w490 w492 w590 w595 w597] -> w405
      tunnel: w404 -> [_ w422 _ _ _ _ _ _ _]
      frame "---------- Framework Operations ----------" {
        # "Dummy case to add a seperator in the Case Structure menu"
      }
      frame "", "Idle" {
        n237 = stacked-sequence {
          frame #0 {
            n238 = control-ref of="Enable Main Pump 2"() -> (w435:refnum<vi>)
            n239 = control-ref of="Drain System to Tree 4"() -> (w429:refnum<vi>)
            n240 = control-ref of="Enable Main Pump"() -> (w428:refnum<vi>)
            n241 = control-ref of="Drain System to Tree 1"() -> (w425:refnum<vi>)
            n242 = control-ref of="Enable Main Pump 4"() -> (w431:refnum<vi>)
            n243 = control-ref of="Drain System to Tree 2"() -> (w434:refnum<vi>)
            n244 = call "GrayOutButtonFromPSPVar.vi"("shared variable refnum in"=refnum<k21> "ni.var.psp://z004551/CDL0100 ReadWriteTags/HMI_Drain_BTank4", "Boolean in"=w431) -> ()  [unwired: 10 in]
            n245 = call "GrayOutButtonFromPSPVar.vi"("shared variable refnum in"=refnum<k21> "ni.var.psp://z004551/CDL0100 ReadWriteTags/HMI_Drain_BTank2", "Boolean in"=w435) -> ()  [unwired: 10 in]
            n246 = call "GrayOutButtonFromPSPVar.vi"("shared variable refnum in"=refnum<k21> "ni.var.psp://z004551/CDL0100 ReadWriteTags/HMI_Drain_BTank1", "Boolean in"=w428) -> ()  [unwired: 10 in]
            n247 = call "GrayOutButtonFromPSPVar.vi"("shared variable refnum in"=refnum<k21> "ni.var.psp://z004551/CDL0100 ReadWriteTags/HMI_Enable_BTnk4_Pump", "Boolean in"=w429) -> ()  [unwired: 10 in]
            n248 = call "GrayOutButtonFromPSPVar.vi"("shared variable refnum in"=refnum<k21> "ni.var.psp://z004551/CDL0100 ReadWriteTags/HMI_Enable_BTnk1_Pump", "Boolean in"=w425) -> ()  [unwired: 10 in]
            n249 = call "GrayOutButtonFromPSPVar.vi"("shared variable refnum in"=refnum<k21> "ni.var.psp://z004551/CDL0100 ReadWriteTags/HMI_Enable_BTnk2_Pump", "Boolean in"=w434) -> ()  [unwired: 10 in]
          }
          frame #1 {
            n250 = control-ref of="Enable Main Pump 3"() -> (w437:refnum<vi>)
            n251 = control-ref of="Drain System to Tree 3"() -> (w439:refnum<vi>)
            n252 = call "GrayOutButtonFromPSPVar.vi"("shared variable refnum in"=refnum<k21> "ni.var.psp://z004551/CDL0100 ReadWriteTags/HMI_Drain_BTank3", "Boolean in"=w437) -> ()  [unwired: 10 in]
            n253 = call "GrayOutButtonFromPSPVar.vi"("shared variable refnum in"=refnum<k21> "ni.var.psp://z004551/CDL0100 ReadWriteTags/HMI_Enable_BTnk3_Pump", "Boolean in"=w439) -> ()  [unwired: 10 in]
          }
          frame #2 {
            n254 = shared-variable-read(refnum<k21> "ni.var.psp://z004551/CDL0100 ReadWriteTags/HMI_Tank4_Enable" ("shared variable refnum in"), FALSE) -> (w449:bool)  [unwired: 1 in, 3 out]
            n255 = shared-variable-read(refnum<k21> "ni.var.psp://z004551/CDL0100 ReadWriteTags/HMI_Tank3_Enable" ("shared variable refnum in"), FALSE) -> (w450:bool)  [unwired: 1 in, 3 out]
            n256 = shared-variable-read(refnum<k21> "ni.var.psp://z004551/CDL0100 ReadWriteTags/HMI_Tank6_Enable" ("shared variable refnum in"), FALSE) -> (w442:bool)  [unwired: 1 in, 3 out]
            n257 = shared-variable-read(refnum<k21> "ni.var.psp://z004551/CDL0100 ReadWriteTags/HMI_Tank5_Enable" ("shared variable refnum in"), FALSE) -> (w443:bool)  [unwired: 1 in, 3 out]
            n258 = shared-variable-read(refnum<k21> "ni.var.psp://z004551/CDL0100 ReadWriteTags/HMI_Tank2_Enable" ("shared variable refnum in"), FALSE) -> (w456:bool)  [unwired: 1 in, 3 out]
            n259 = shared-variable-read(refnum<k21> "ni.var.psp://z004551/CDL0100 ReadWriteTags/HMI_Tank1_Enable" ("shared variable refnum in"), FALSE) -> (w457:bool)  [unwired: 1 in, 3 out]
            n260 = Or(x=w450, y=w449) -> (x .or. y?=→"Plating Tanks In Use S. PE":bool)
            n261 = Or(x=w443, y=w442) -> (x .or. y?=→"Plating Tanks In Use S. PE 3":bool)
            n262 = Or(x=w457, y=w456) -> (x .or. y?=→"Plating Tanks In Use South PE":bool)
          }
          frame #3 {
            n263 = shared-variable-read(refnum<k21> "ni.var.psp://z004551/CDL0100 ReadWriteTags/HMI_BAS_Proc2_AddDIVolume" ("shared variable refnum in"), FALSE) -> (w467:bool)  [unwired: 1 in, 3 out]
            n264 = shared-variable-read(refnum<k21> "ni.var.psp://z004551/CDL0100 ReadWriteTags/HMI_BAS_Proc3_AddDIVolume" ("shared variable refnum in"), FALSE) -> (w463:bool)  [unwired: 1 in, 3 out]
            n265 = call <userlib>:"Boolean Trigger__ogtk.vi"("Boolean Input"=w467) -> ("Falling Edge"=w466:bool)  [unwired: 1 in, 1 out]
            n266 = call <userlib>:"Boolean Trigger__ogtk.vi"("Boolean Input"=w463) -> ("Falling Edge"=w462:bool)  [unwired: 1 in, 1 out]
            n267 = case shown="True" w462 {
              frame False {
              }
              frame True {
                n268 = local write "Add DI water 3"(FALSE ("Add DI water 3")) -> ()
              }
            }
            n269 = case shown="True" w466 {
              frame False {
              }
              frame True {
                n270 = local write "Add DI water 2"(FALSE ("Add DI water 2")) -> ()
              }
            }
          }
          frame #4 {
            n271 = shared-variable-read(refnum<k21> "ni.var.psp://z004551/CDL0100 ReadWriteTags/HMI_BAS_Proc1_AddDIVolume" ("shared variable refnum in"), FALSE) -> (w473:bool)  [unwired: 1 in, 3 out]
            n272 = shared-variable-read(refnum<k21> "ni.var.psp://z004551/CDL0100 ReadWriteTags/HMI_BAS_Proc4_AddDIVolume" ("shared variable refnum in"), FALSE) -> (w477:bool)  [unwired: 1 in, 3 out]
            n273 = call <userlib>:"Boolean Trigger__ogtk.vi"("Boolean Input"=w473) -> ("Falling Edge"=w472:bool)  [unwired: 1 in, 1 out]
            n274 = call <userlib>:"Boolean Trigger__ogtk.vi"("Boolean Input"=w477) -> ("Falling Edge"=w476:bool)  [unwired: 1 in, 1 out]
            n275 = case shown="True" w476 {
              frame False {
              }
              frame True {
                n276 = local write "Add DI water 4"(FALSE ("Add DI water 4")) -> ()
              }
            }
            n277 = case shown="True" w472 {
              frame False {
              }
              frame True {
                n278 = local write "Add DI water 1"(FALSE ("Add DI water 1")) -> ()
              }
            }
          }
        }
        n279 = call <userlib>:"TAE Alarm Engine.vi"("AE_CommIn"=w423, "Alarm List"=w422) -> ("Alarm queue out"=w421:T11)  [unwired: 7 in, 2 out]
        n280 = control-ref of="status"() -> (w420:refnum<vi>)
        n281 = call <userlib>:"TAE Format Alarm Ticker.vi"("Alarm Ticker Ref"=w420) -> ()  [unwired: 15 in]
        n282 = control-ref of="Alarms"() -> (w419:refnum<vi>)
        n283 = call <userlib>:"TAE Format Active Alarm Display.vi"("List Box Ref"=w419) -> ()  [unwired: 14 in, 1 out]
      }
      frame "Missing Message Handler", Default {
        # "Call this case if a message is received that is not handled \nby any other case. Typically this is a programming error\nas a result of a typo or unhandled message/missing message handler."
        n284 = Format Into String(format string="DevError: Missing message handler for '%s\" message." ("message"), w485) -> (resulting string=w483:string)  [unwired: 2 in, 1 out]
        n285 = One Button Dialog(message=w483) -> ()  [unwired: 2 out]
      }
      frame "Error" {
        # "General Error Case - this case is called if an error is passed using the error cluster below. Typically most new errors should be handed in each individual case and not passed in the rror cluster. If necessary a custom error handler case should be added and called from other cases."
        n286 = call <vilib>:"Simple Error Handler.vi"("error in (no error)"=w488) -> ()  [unwired: 1 in, 8 out]
      }
      frame "---------- Generic Operations ----------" {
        # "Dummy case to add a seperator in the Case Structure menu"
      }
      frame "Initialize" {
        n287 = stacked-sequence {
          tunnel: w494 -> [w507 _ _ _ _ _]
          tunnel: [w504 _ _ _ _ _] -> w493
          frame #0 {
            n288 = shared-variable-read(refnum<k21> "ni.var.psp://z004551/CDL0100 ReadWriteTags/HMI_Enable_BTnk1_Pump" ("shared variable refnum in"), FALSE) -> (w501:bool)  [unwired: 1 in, 3 out]
            n289 = shared-variable-read(refnum<k21> "ni.var.psp://z004551/CDL0100 ReadWriteTags/HMI_Run" ("shared variable refnum in"), w507, FALSE) -> (w504:errorcluster, w505:bool)  [unwired: 2 out]
            n290 = local write "Enable Main Pump"(w501) -> ()
            n291 = local write "Run"(w505) -> ()
            n292 = shared-variable-read(refnum<k21> "ni.var.psp://z004551/CDL0100 ReadWriteTags/HMI_Proc1_OxFlow_SetPnt" ("shared variable refnum in"), 0.0) -> (w495:dbl)  [unwired: 1 in, 3 out]
            n293 = shared-variable-read(refnum<k21> "ni.var.psp://z004551/CDL0100 ReadWriteTags/HMI_Drain_BTank1" ("shared variable refnum in"), FALSE) -> (w498:bool)  [unwired: 1 in, 3 out]
            n294 = local write "Drain System to Tree 1"(w498) -> ()
            n295 = local write "Flow to Oxide 1"(w495) -> ()
          }
          frame #1 {
            n296 = shared-variable-read(refnum<k21> "ni.var.psp://z004551/CDL0100 ReadWriteTags/HMI_Drain_BTank2" ("shared variable refnum in"), FALSE) -> (w524:bool)  [unwired: 1 in, 3 out]
            n297 = shared-variable-read(refnum<k21> "ni.var.psp://z004551/CDL0100 ReadWriteTags/HMI_Proc2_Run_OxideSys" ("shared variable refnum in"), FALSE) -> (w518:bool)  [unwired: 1 in, 3 out]
            n298 = shared-variable-read(refnum<k21> "ni.var.psp://z004551/CDL0100 ReadWriteTags/HMI_Proc2_OxFlow_SetPnt" ("shared variable refnum in"), 0.0) -> (w515:dbl)  [unwired: 1 in, 3 out]
            n299 = shared-variable-read(refnum<k21> "ni.var.psp://z004551/CDL0100 ReadWriteTags/HMI_BAS_TNK2_T_Setpoint" ("shared variable refnum in"), 0.0) -> (w512:dbl)  [unwired: 1 in, 3 out]
            n300 = shared-variable-read(refnum<k21> "ni.var.psp://z004551/CDL0100 ReadWriteTags/HMI_BAS_Proc2_AddDIVolume" ("shared variable refnum in"), FALSE) -> (w509:bool)  [unwired: 1 in, 3 out]
            n301 = shared-variable-read(refnum<k21> "ni.var.psp://z004551/CDL0100 ReadWriteTags/HMI_Enable_BTnk2_Pump" ("shared variable refnum in"), FALSE) -> (w527:bool)  [unwired: 1 in, 3 out]
            n302 = shared-variable-read(refnum<k21> "ni.var.psp://z004551/CDL0100 ReadWriteTags/HMI_BAS_Tank2_TControl_Enable" ("shared variable refnum in"), FALSE) -> (w521:bool)  [unwired: 1 in, 3 out]
            n303 = local write "Drain System to Tree 2"(w524) -> ()
            n304 = local write "Flow to Oxide 2"(w515) -> ()
            n305 = local write "Enable Oxide System 2"(w518) -> ()
            n306 = local write "Add DI water 2"(w509) -> ()
            n307 = local write "Enable T Control 2"(w521) -> ()
            n308 = local write "Enable Main Pump 2"(w527) -> ()
            n309 = local write "T Setpoint 2"(w512) -> ()
          }
          frame #2 {
            n310 = shared-variable-read(refnum<k21> "ni.var.psp://z004551/CDL0100 ReadWriteTags/HMI_BAS_Tank1_TControl_Enable" ("shared variable refnum in"), FALSE) -> (w533:bool)  [unwired: 1 in, 3 out]
            n311 = shared-variable-read(refnum<k21> "ni.var.psp://z004551/CDL0100 ReadWriteTags/HMI_Proc1_CuOxideAddAmnt" ("shared variable refnum in"), 0.0) -> (w530:dbl)  [unwired: 1 in, 3 out]
            n312 = shared-variable-read(refnum<k21> "ni.var.psp://z004551/CDL0100 ReadWriteTags/HMI_BAS_Proc2_DI_Setpnt" ("shared variable refnum in"), 0.0) -> (w545:dbl)  [unwired: 1 in, 3 out]
            n313 = shared-variable-read(refnum<k21> "ni.var.psp://z004551/CDL0100 ReadWriteTags/HMI_BAS_TNK1_T_Setpoint" ("shared variable refnum in"), 0.0) -> (w536:dbl)  [unwired: 1 in, 3 out]
            n314 = shared-variable-read(refnum<k21> "ni.var.psp://z004551/CDL0100 ReadWriteTags/HMI_BAS_Proc1_DI_Setpnt" ("shared variable refnum in"), 0.0) -> (w543:dbl)  [unwired: 1 in, 3 out]
            n315 = shared-variable-read(refnum<k21> "ni.var.psp://z004551/CDL0100 ReadWriteTags/HMI_BAS_Proc1_AddDIVolume" ("shared variable refnum in"), FALSE) -> (w544:bool)  [unwired: 1 in, 3 out]
            n316 = local write "Oxide grams to Add 1"(w530) -> ()
            n317 = local write "DI Add Volume 2"(w545) -> ()
            n318 = local write "Enable T Control 1"(w533) -> ()
            n319 = local write "Add DI water 1"(w544) -> ()
            n320 = local write "DI Add Volume 1"(w543) -> ()
            n321 = local write "T Setpoint 1"(w536) -> ()
          }
          frame #3 {
            n322 = shared-variable-read(refnum<k21> "ni.var.psp://z004551/CDL0100 ReadWriteTags/HMI_BAS_Tank3_TControl_Enable" ("shared variable refnum in"), FALSE) -> (w554:bool)  [unwired: 1 in, 3 out]
            n323 = shared-variable-read(refnum<k21> "ni.var.psp://z004551/CDL0100 ReadWriteTags/HMI_BAS_Proc3_AddDIVolume" ("shared variable refnum in"), FALSE) -> (w548:bool)  [unwired: 1 in, 3 out]
            n324 = shared-variable-read(refnum<k21> "ni.var.psp://z004551/CDL0100 ReadWriteTags/HMI_Enable_BTnk3_Pump" ("shared variable refnum in"), FALSE) -> (w562:bool)  [unwired: 1 in, 3 out]
            n325 = shared-variable-read(refnum<k21> "ni.var.psp://z004551/CDL0100 ReadWriteTags/HMI_BAS_Proc3_DI_Setpnt" ("shared variable refnum in"), 0.0) -> (w551:dbl)  [unwired: 1 in, 3 out]
            n326 = shared-variable-read(refnum<k21> "ni.var.psp://z004551/CDL0100 ReadWriteTags/HMI_Drain_BTank3" ("shared variable refnum in"), FALSE) -> (w561:bool)  [unwired: 1 in, 3 out]
            n327 = shared-variable-read(refnum<k21> "ni.var.psp://z004551/CDL0100 ReadWriteTags/HMI_BAS_TNK3_T_Setpoint" ("shared variable refnum in"), 0.0) -> (w557:dbl)  [unwired: 1 in, 3 out]
            n328 = local write "Drain System to Tree 3"(w561) -> ()
            n329 = local write "Enable Main Pump 3"(w562) -> ()
            n330 = local write "Add DI water 3"(w548) -> ()
            n331 = local write "DI Add Volume 3"(w551) -> ()
            n332 = local write "T Setpoint 3"(w557) -> ()
            n333 = local write "Enable T Control 3"(w554) -> ()
          }
          frame #4 {
            n334 = shared-variable-read(refnum<k21> "ni.var.psp://z004551/CDL0100 ReadWriteTags/HMI_Proc1_Run_OxideSys" ("shared variable refnum in"), FALSE) -> (w566:bool)  [unwired: 1 in, 3 out]
            n335 = shared-variable-read(refnum<k21> "ni.var.psp://z004551/CDL0100 ReadWriteTags/HMI_Proc3_Run_OxideSys" ("shared variable refnum in"), FALSE) -> (w570:bool)  [unwired: 1 in, 3 out]
            n336 = shared-variable-read(refnum<k21> "ni.var.psp://z004551/CDL0100 ReadWriteTags/HMI_Proc3_OxFlow_SetPnt" ("shared variable refnum in"), 0.0) -> (w569:dbl)  [unwired: 1 in, 3 out]
            n337 = local write "Flow to Oxide 3"(w569) -> ()
            n338 = local write "Enable Oxide System 3"(w570) -> ()
            n339 = local write "Enable Oxide System 1"(w566) -> ()
          }
          frame #5 {
            n340 = shared-variable-read(refnum<k21> "ni.var.psp://z004551/CDL0100 ReadWriteTags/HMI_BAS_Tnk4RecircPmpPcnt" ("shared variable refnum in"), 0.0) -> (w575:dbl)  [unwired: 1 in, 3 out]
            n341 = shared-variable-read(refnum<k21> "ni.var.psp://z004551/CDL0100 ReadWriteTags/HMI_Enable_BTnk4_Pump" ("shared variable refnum in"), FALSE) -> (w584:bool)  [unwired: 1 in, 3 out]
            n342 = shared-variable-read(refnum<k21> "ni.var.psp://z004551/CDL0100 ReadWriteTags/HMI_BAS_Proc4_AddDIVolume" ("shared variable refnum in"), FALSE) -> (w578:bool)  [unwired: 1 in, 3 out]
            n343 = shared-variable-read(refnum<k21> "ni.var.psp://z004551/CDL0100 ReadWriteTags/HMI_Drain_BTank4" ("shared variable refnum in"), FALSE) -> (w585:bool)  [unwired: 1 in, 3 out]
            n344 = shared-variable-read(refnum<k21> "ni.var.psp://z004551/CDL0100 ReadWriteTags/HMI_BAS_Proc4_DI_Setpnt" ("shared variable refnum in"), 0.0) -> (w579:dbl)  [unwired: 1 in, 3 out]
            n345 = local write "Pump Speed 4"(w575) -> ()
            n346 = local write "DI Add Volume 4"(w579) -> ()
            n347 = local write "Add DI water 4"(w578) -> ()
            n348 = local write "Enable Main Pump 4"(w584) -> ()
            n349 = local write "Drain System to Tree 4"(w585) -> ()
          }
        }
      }
      frame "Exit" {
        # "Destroy message queue >> this will halt the UI event handler loop"
        # "Stop the VI\n>> Perform any cleanup tasks in this message case.\n>> Clear display before closing."
        n350 = call <vilib>:"Destroy Message Queue.vi"("message queue in"=w592, "error in"=w593) -> ("error out"=w591:errorcluster)  [unwired: 11 in, 2 out]
        n351 = local write "status"("" ("Status")) -> ()
      }
      frame "---------- Application Operations ----------" {
        # "Dummy case to add a seperator in the Case Structure menu"
      }
      frame "Write_Tag" {
        n352 = call-poly <vilib>:"Write Message.vi"("error in"=w600, "data"=w598, "name"="WriteTag", "connection info in"=w601) -> ("error out"=w599:errorcluster)  [unwired: 6 in, 1 out]
      }
    }
  }
  n353 = call-poly <vilib>:"Get Connection Reference.vi"("error in"=w24, "connection info in"=w22) -> ("error out"=w27:errorcluster, "connection ID out"=w26:refnum<k5>)  [unwired: 8 out]
  n354 = TCP Close Connection(connection ID=w26, error in (no error)=w27) -> (error out=w29:errorcluster)  [unwired: 2 out]
  n355 = call <userlib>:"TAE Close.vi"("Alarm queue out"=w12) -> ()  [unwired: 10 in, 1 out]
  n356 = call <vilib>:"Error to Warning.vi"("1st Error to Convert"=w28, "error in"=w29) -> ("warning out"=w25:errorcluster)  [unwired: 3 in, 10 out]
  n357 = call <vilib>:"Simple Error Handler.vi"("error in (no error)"=w25) -> ()  [unwired: 4 in, 5 out]
